vi "PhidgetAddServer.vi"(5 "Password":string, 7 "Host":string, 8 "error in":errorcluster, 9 "Flags":i32, 10 "Port":i32, 11 "Name":string) -> (0 "error out":errorcluster)   [LabVIEW 2012, in "Phidget Common.lvlib"]
doc: "${AddServer:Header}"
uses:
  <instrlib>/Phidgets/Phidget Common/Phidget Common.lvlib
  phidget22.dll
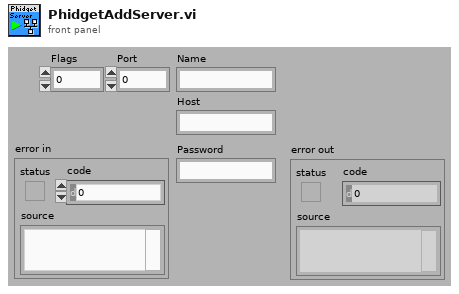
[diagram p1: front panel]
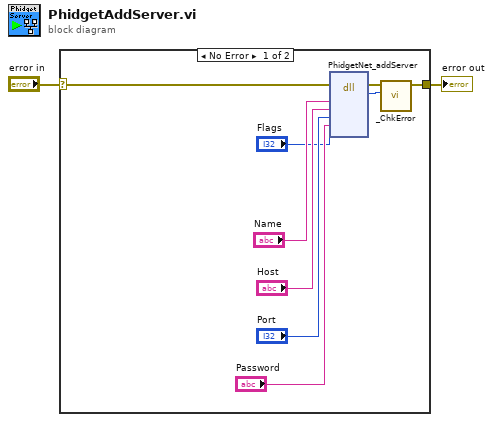
[diagram p0: block diagram]
diagram:
  n1 = case shown="No Error" "error in" {
    selector: "error in" -> [w6 w12]
    tunnel: [w4 w12] -> w1
    frame No Error {
      n2 = dll-call lib="phidget22.dll" fn="PhidgetNet_addServer"(error in=w6, "name"="Name", "host"="Host", "port"="Port", "passwd"="Password", "flags"="Flags") -> (error out=w5:errorcluster, "return type"=w11:i32)  [unwired: 7 in, 1 out]
      n3 = call <instrlib>:"_ChkError.vi"("Return Code"=w11, "error in (no error)"=w5) -> ("error out"=w4:errorcluster)  [unwired: 9 in]
    }
    frame Error {
    }
  }
  "error out" <- w1
